vi "PitScout.vi"() -> ()   [LabVIEW 2015]
uses:
  <vilib>/Utility/sysdir.llb/System Directory Type.ctl
panel:
  in  "stop":bool
  in  "What Kind of Robot do they consider themselves?":string(combo)
  in  "Can they scale the tower?":string(combo)
  in  "Team Number":string
  in  "Best attribute about their robot?":string
  in  "High Goal, Low Goal, or Both?":string
  in  "Which defences can they go through?":string
  in  "Do they have an Autonomous and what does it do?":string
  in  "What Kind of Drive Train?":string
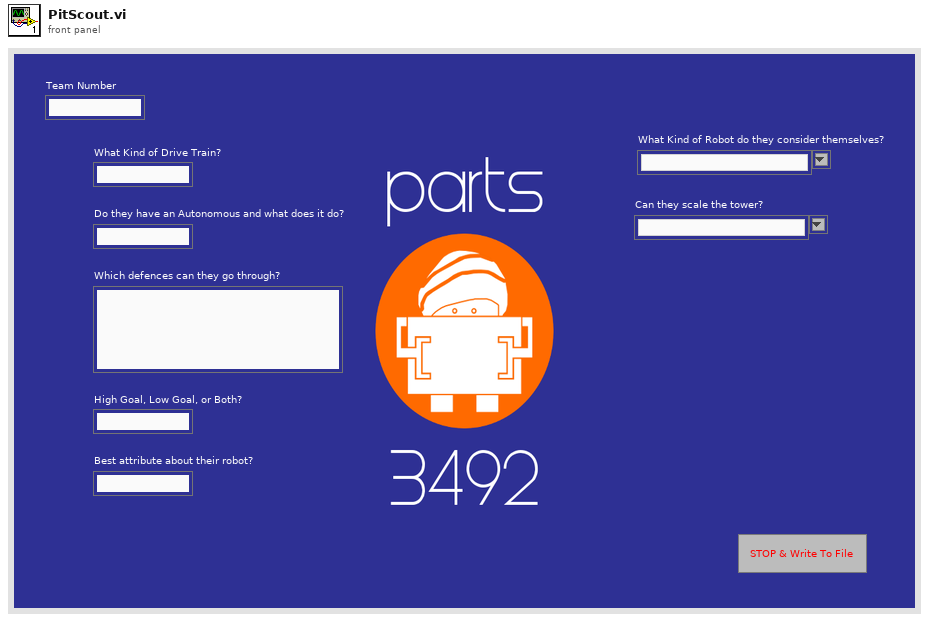
[diagram p1: front panel]
types:
  T1 = typedef "System Directory Type.ctl" = i32
  T2 = enum16{"open", "replace", "create", "open or create", "replace or create", "replace or create with confirmation"}
  T3 = enum32{"invalid app kind", "Development System", "Run Time System", "Student Edition", "Embedded LabVIEW", "Evaluation", "Custom"}
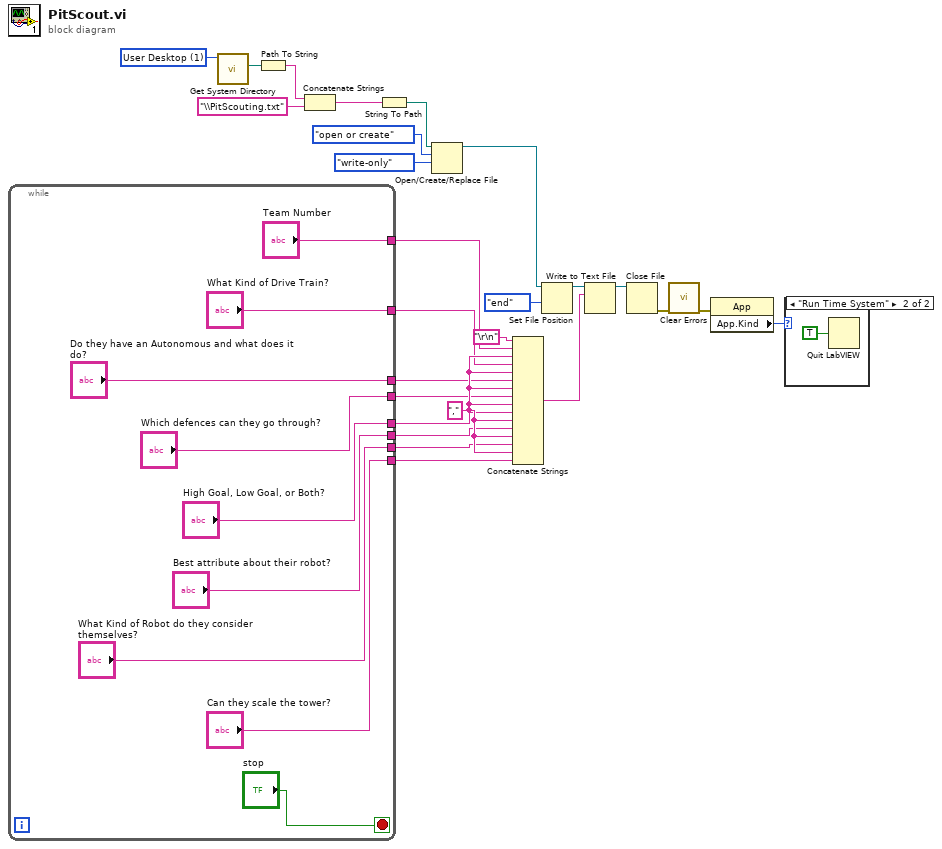
[diagram p0: block diagram]
diagram:
  w12 = T1 1 items=["User Home"=0, "User Desktop"=1, "User Documents"=2, "User Application Data"=3, "User Preferences"=4, "User Temporary"=5, "Public Documents"=6, "Public Application Data"=7, "Public Preferences"=8, "Public Cache"=13, "System Core Libraries"=9, "System Installed Libraries"=10, "Application Files"=11, "Boot Volume Root"=12] ("system directory type")
  w25 = "," ("string")
  n1 = while {
    tunnel: ["Team Number"] -> w26
    tunnel: ["What Kind of Drive Train?"] -> w24
    tunnel: ["Do they have an Autonomous and what does it do?"] -> w23
    tunnel: ["Which defences can they go through?"] -> w22
    tunnel: ["High Goal, Low Goal, or Both?"] -> w21
    tunnel: ["Best attribute about their robot?"] -> w20
    tunnel: ["What Kind of Robot do they consider themselves?"] -> w19
    tunnel: ["Can they scale the tower?"] -> w18
    stop <- "stop" stop-if-true
  }
  n2 = call <vilib>:"Get System Directory.vi"("system directory type"=w12) -> ("system directory"=w11:path)  [unwired: 10 in]
  n3 = Path To String(path=w11) -> (string=w10:string)
  n4 = Concatenate Strings(w10, "\\PitScouting.txt" ("string")) -> (w8:string)
  n5 = String To Path(string=w8) -> (path=w7:path)
  n6 = Open/Create/Replace File(file path (use dialog)=w7, operation (0:open)=T2."open or create", access (0:read/write)=enum16{"read/write", "read-only", "write-only"}."write-only") -> (refnum out=w14:refnum<file>)  [unwired: 3 in, 2 out]
  n7 = Concatenate Strings("\r\n", w26, w25, w24, w25, w23, w25, w22, w25, w21, w25, w20, w25, w19, w25, w18) -> (w1:string)
  n8 = Set File Position(refnum=w14, from (0:start)=enum16{"start", "end", "current"}."end") -> (refnum out=w2:refnum<file>)  [unwired: 2 in, 1 out]
  n9 = Write to Text File(file (use dialog)=w2, text=w1) -> (refnum out=w6:refnum<file>)  [unwired: 2 in, 2 out]
  n10 = Close File(refnum=w6) -> (error out=w5:errorcluster)  [unwired: 1 in, 1 out]
  n11 = call <vilib>:"Clear Errors.vi"("error in (no error)"=w5) -> ("error out"=w4:errorcluster)  [unwired: 5 in, 1 out]
  n12 = property class="App"(error in=w4) -> ("App.Kind"=w3:T3)  [unwired: 1 in, 2 out]
  n13 = case shown="\"Run Time System\"" w3 {
    frame Default {
    }
    frame "Run Time System" {
      n14 = Quit LabVIEW(quit? (T)=TRUE) -> ()
    }
  }
